vi "IncrementBlueSerializableVerPathWrapperWrapper.vi"(7 "Application":refnum<vi>, 8 "error in (no error)":errorcluster, 9 "Version Bump 2":T1, 10 "Version Bump 1":T1, 11 "LVClass name":string) -> (0 "error out":errorcluster, 3 "BlueSerializableVersion":u16)   [LabVIEW 2019, in "BlueSerializationScripts.lvlib"]
uses:
  BlueSerializationScripts.lvlib
  <vilib>/Utility/EditLVLibs/LibVersion.ctl
  UserAppLibs/IncrementMutationHistory/IncrementMutationHistory.lvlib
  <vilib>/Utility/EditLVLibs/Edit LVLibs.lvlib
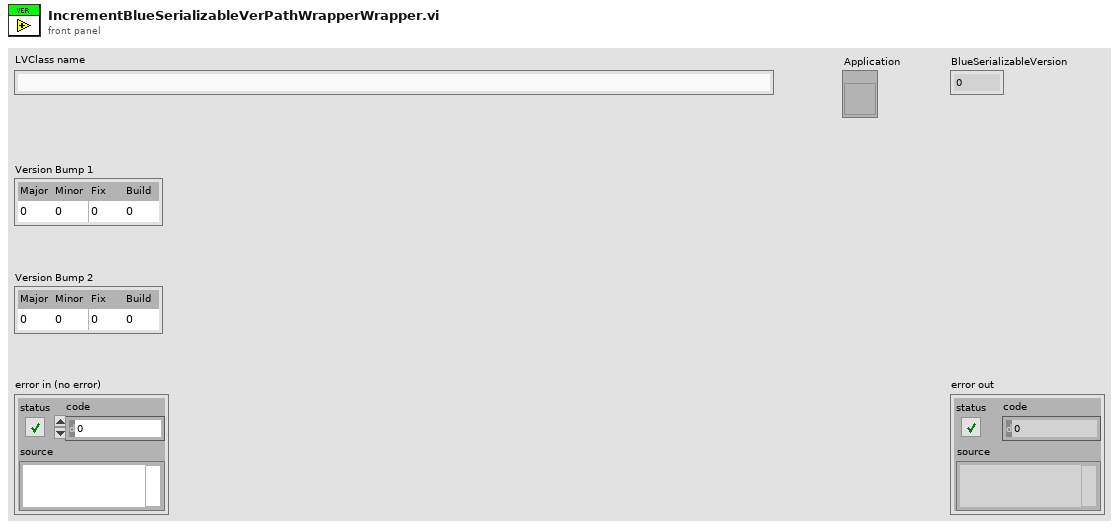
[diagram p1: front panel]
types:
  T1 = typedef "Edit LVLibs.lvlib/LibVersion.ctl" = cluster{"Major":u16, "Minor":u16, "Fix":u16, "Build":u16}
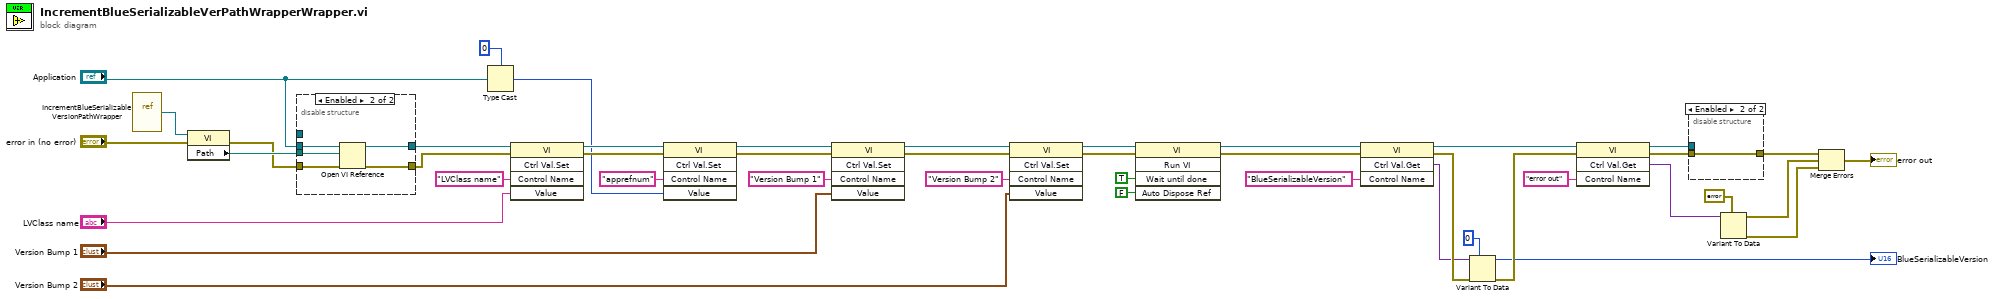
[diagram p0: block diagram]
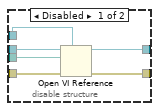
[diagram p2: hidden frame]
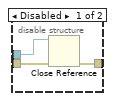
[diagram p3: hidden frame]
diagram:
  n1 = vi-ref "IncrementBlueSerializableVersionPathWrapper.vi"() -> (w44:refnum<vi>)
  n2 = property class="VI"(reference=w44, error in="error in (no error)") -> (error out=w42:errorcluster, "Path"=w43:path)  [unwired: 1 out]
  n3 = disable-structure shown="Enabled" {
    disable-tunnel: w43 -> [w50 w54]
    disable-tunnel: _ -> [w49 _]
    disable-tunnel: w42 -> [w48 w55]
    disable-tunnel: [w47 w52] -> w2
    disable-tunnel: [w46 w51] -> w1
    disable-tunnel: "Application" -> [w45 w53]
    frame Disabled {
      n4 = Open VI Reference(type specifier VI Refnum (for type only)=w49, application reference (local)=w45, vi path=w50, error in (no error)=w48) -> (vi reference=w47:refnum<vi>, error out=w46:errorcluster)  [unwired: 2 in]
    }
    frame Enabled {
      n5 = Open VI Reference(application reference (local)=w53, vi path=w54, error in (no error)=w55) -> (vi reference=w52:refnum<vi>, error out=w51:errorcluster)  [unwired: 3 in]
    }
  }
  n6 = Type Cast(type=u32 0 ("apprefnum"), x="Application") -> (*(type *) &x=w3:u32)
  n7 = invoke class="VI" method="Ctrl Val.Set"(reference=w2, error in=w1, "Control Name"="LVClass name", "Value"="LVClass name") -> (reference out=w8:refnum<vi>, error out=w9:errorcluster)  [unwired: 1 in, 3 out]
  n8 = invoke class="VI" method="Ctrl Val.Set"(reference=w8, error in=w9, "Control Name"="apprefnum", "Value"=w3) -> (reference out=w7:refnum<vi>, error out=w6:errorcluster)  [unwired: 1 in, 3 out]
  n9 = invoke class="VI" method="Ctrl Val.Set"(reference=w7, error in=w6, "Control Name"="Version Bump 1", "Value"="Version Bump 1") -> (reference out=w20:refnum<vi>, error out=w19:errorcluster)  [unwired: 1 in, 3 out]
  n10 = invoke class="VI" method="Ctrl Val.Set"(reference=w20, error in=w19, "Control Name"="Version Bump 2", "Value"="Version Bump 2") -> (reference out=w15:refnum<vi>, error out=w14:errorcluster)  [unwired: 1 in, 3 out]
  n11 = invoke class="VI" method="Run VI"(reference=w15, error in=w14, "Wait until done"=TRUE ("Wait Until Done"), "Auto Dispose Ref"=FALSE ("Auto Dispose Reference")) -> (reference out=w38:refnum<vi>, error out=w34:errorcluster)  [unwired: 1 in, 3 out]
  n12 = invoke class="VI" method="Ctrl Val.Get"(reference=w38, error in=w34, "Control Name"="BlueSerializableVersion") -> (reference out=w35:refnum<vi>, error out=w33:errorcluster, "Get Control Value Variant"=w32:variant)  [unwired: 1 in, 1 out]
  n13 = Variant To Data(error in=w33, type=u16 0 ("BlueSerializableVersion"), Variant=w32) -> (data=→"BlueSerializableVersion":u16, error out=w31:errorcluster)
  n14 = invoke class="VI" method="Ctrl Val.Get"(reference=w35, error in=w31, "Control Name"="error out") -> (reference out=w24:refnum<vi>, error out=w26:errorcluster, "Get Control Value Variant"=w30:variant)  [unwired: 1 in, 1 out]
  n15 = disable-structure shown="Enabled" {
    disable-tunnel: w26 -> [w58 w59]
    disable-tunnel: [w57 w59] -> w25
    disable-tunnel: w24 -> [w56 _]
    frame Disabled {
      n16 = Close Reference(reference=w56, error in (no error)=w58) -> (error out=w57:errorcluster)
    }
    frame Enabled {
    }
  }
  n17 = Variant To Data(type=errorcluster {"status"=FALSE, "code"=0, "source"=""} ("error out"), Variant=w30) -> (data=w28:errorcluster, error out=w27:errorcluster)  [unwired: 1 in]
  n18 = Merge Errors(w25, w28, w27) -> (→"error out":errorcluster)
